vi "LoadSavedQueue.vi"(0 "Program Interface in":refnum<class "Program Interface.lvclass">, 5 "error in (no error)":errorcluster) -> (14 "Program Interface out":refnum<class "Program Interface.lvclass">, 19 "error out":errorcluster)   [LabVIEW 2019, in "Program Interface.lvclass"]
uses:
  Program Interface.lvclass
  Program Interface.lvclass/Program Interface.ctl
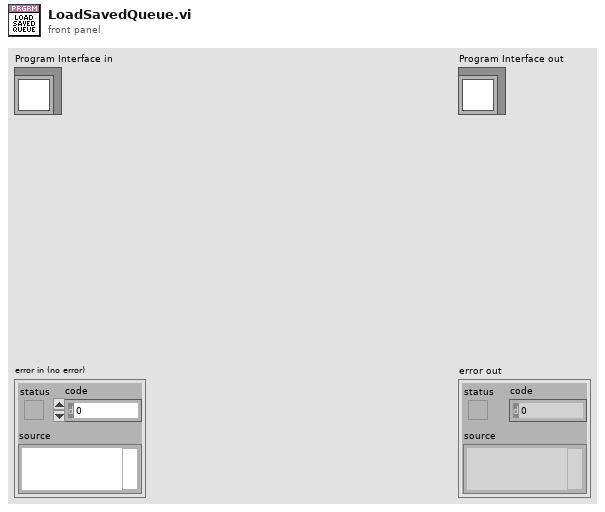
[diagram p1: front panel]
types:
  T1 = typedef "Program Interface.lvclass/SavedQueue.ctl" = cluster{"Name":string, "Programs":string[]}
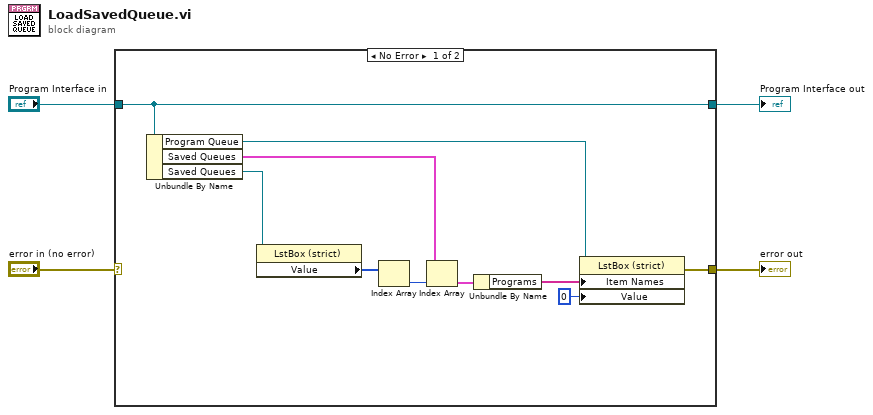
[diagram p0: block diagram]
diagram:
  n1 = case shown="No Error" "error in (no error)" {
    selector: "error in (no error)" -> [_ w16]
    tunnel: [w7 w16] -> w3
    tunnel: [w5 w15] -> w1
    tunnel: "Program Interface in" -> [w5 w15]
    frame No Error {
      n2 = Unbundle By Name(w5) -> ("Program Queue"=w10:refnum<vi>, "Saved Queues"=w14:T1[], "Saved Queues"=w11:refnum<vi>)
      n3 = property class="LstBox (strict)"(reference=w11) -> ("Value"=w13:i32[])  [unwired: 1 in, 2 out]
      n4 = Index Array(array=w13) -> (element=w12:i32)  [unwired: 1 in]
      n5 = Index Array(array=w14, index=w12) -> (element=w9:T1)
      n6 = Unbundle By Name(w9) -> ("Programs"=w8:string[])
      n7 = property class="LstBox (strict)"(reference=w10, "Item Names"=w8, "Value"=0) -> (error out=w7:errorcluster)  [unwired: 1 in, 1 out]
    }
    frame Error {
    }
  }
  "error out" <- w3
  "Program Interface out" <- w1
